vi "CTRE_Phoenix_CANcoder_GetMagnetFieldStrength.vi"(0 "CTRE_CANcoder_DeviceRef":T2, 11 "error in":errorcluster) -> (4 "CTRE_CANcoder_DeviceRef":T2, 6 "Magnet Field Strength":T1, 15 "error out":errorcluster)   [LabVIEW 2020]
doc: "Gets the magnet's health.\n\n<b>Magnet Field Strength</b> is the magnet health code (red/orange/green)."
uses:
  <vilib>/Rock Robotics/WPI/ThirdParty/Phoenix-LabVIEW/CANCoder/Controls/CTRE_Phoenix_CANcoder_DeviceRef.ctl
  <vilib>/Rock Robotics/WPI/ThirdParty/Phoenix-LabVIEW/CANCoder/Controls/CTRE_Phoenix_CANcoder_MagnetFieldStrength.ctl
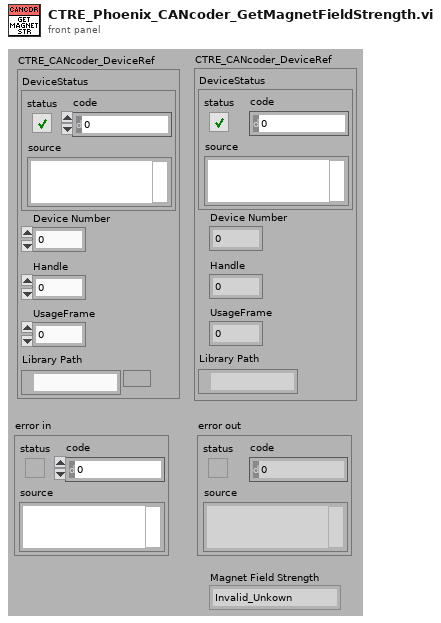
[diagram p1: front panel]
types:
  T1 = typedef "CTRE_Phoenix_CANcoder_MagnetFieldStrength.ctl" = enum16{"Invalid_Unkown", "BadRange_RedLED", "Adequate_OrangeLED", "Good_GreenLED"}
  T2 = typedef "CTRE_Phoenix_CANcoder_DeviceRef.ctl" = cluster{"DeviceStatus":errorcluster, "Device Number":u8, "Handle":u64, "UsageFrame":u32, "Library Path":path}
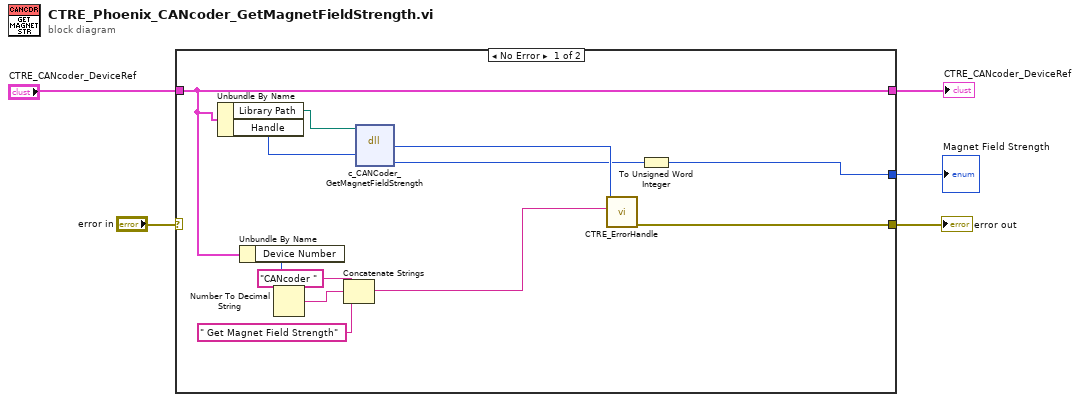
[diagram p0: block diagram]
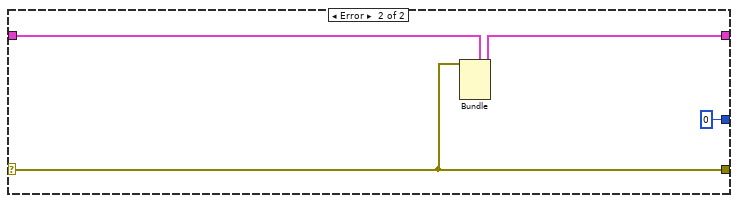
[diagram p2: hidden frame]
diagram:
  n1 = case shown="No Error" "error in" {
    selector: "error in" -> [_ w20]
    tunnel: "CTRE_CANcoder_DeviceRef" -> [w10 w21]
    tunnel: [w17 w20] -> w5
    tunnel: [w10 w19] -> w2
    tunnel: [w6 u16 0] -> w1
    frame No Error {
      n2 = Unbundle By Name(w10) -> ("Library Path"=w9:path, "Handle"=w8:u64)
      n3 = Unbundle By Name(w10) -> ("Device Number"=w13:u8)
      n4 = Number To Decimal String(number=w13) -> (decimal integer string=w15:string)  [unwired: 1 in]
      n5 = Concatenate Strings("CANcoder " ("string"), w15, " Get Magnet Field Strength" ("string")) -> (w11:string)
      n6 = dll-call lib="?" fn="c_CANCoder_GetMagnetFieldStrength"(path in=w9, "handle"=w8) -> ("return type"=w12:i32, "magnetFieldStrength"=w7:i32)  [unwired: 4 in, 2 out]
      n7 = call <vilib>:"CTRE_ErrorHandle.vi"("origin"=w11, "code"=w12) -> ("error out"=w17:errorcluster)  [unwired: 9 in]
      n8 = To Unsigned Word Integer(number=w7) -> (unsigned 16bit integer=w6:u16)
    }
    frame Error {
      n9 = Bundle(cluster=w21, "DeviceStatus"=w20) -> (w19:T2)  [unwired: 4 in]
    }
  }
  "error out" <- w5
  "CTRE_CANcoder_DeviceRef" <- w2
  "Magnet Field Strength" <- w1
